vi "Network Streams Chat Window Launcher.vi"() -> ()   [LabVIEW 2020]
uses:
  Chat Window/Chat Window.lvclass
  C:/Program Files (x86)/National Instruments/LabVIEW 2020/vi.lib/ActorFramework/Actor/Actor.lvclass
  Protocols/Network Stream Strategy/Network Stream/Network Stream.lvclass/Network Stream.ctl
  Protocols/Network Stream Strategy/Network Stream Initiator/Network Stream Initiator.lvclass/Network Stream Initiator.ctl
  Chat Window/Chat Window.lvclass/Chat Window.ctl
  Protocols/Network Stream Strategy/Network Stream/Write Buffer Size.vi
  Protocols/Network Stream Strategy/Network Stream/Write Name.vi
  Protocols/Network Stream Strategy/Network Stream Initiator/Network Stream Initiator.lvclass
  C:/justACS/network-endpoints/4.0/Source/Protocols/Network Stream Strategy/Network Stream/Network Stream.lvclass
  C:/justACS/network-endpoints/4.0/Source/Abstract Classes/Message Stream/Message Stream.lvclass
  Protocols/Network Stream Strategy/Netowrk Stream Listener/Network Stream Listener.lvclass
  <vilib>/ActorFramework/Actor/Actor.lvclass
panel:
  in  "Listener Name":string="Bob"
  in  "Address":string="127.0.0.1"
  in  "Initiator Name":string="Fred"
  out "error out":errorcluster
  # "This VI launches two instances of a chat window actor.  The two chat windows launch nested endpoints, which connect via a Network Stream mesage stream.\n\n1.  (Optional)  Specify the IP address for this machine, and the names of the two stream endpoints\n2.  Run this VI.\n3.  Stop the application by closing either chat window.\n\nAF_Debug_Trace is set to TRUE in this project, so you can follow the action with the Desktop Execution Trace Toolkit."
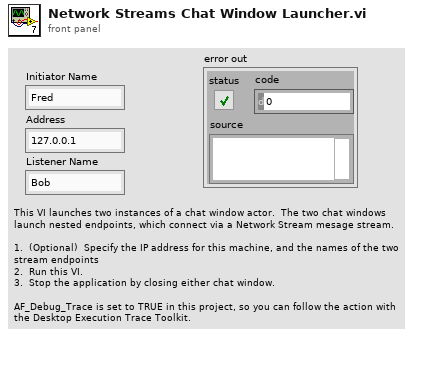
[diagram p1: front panel]
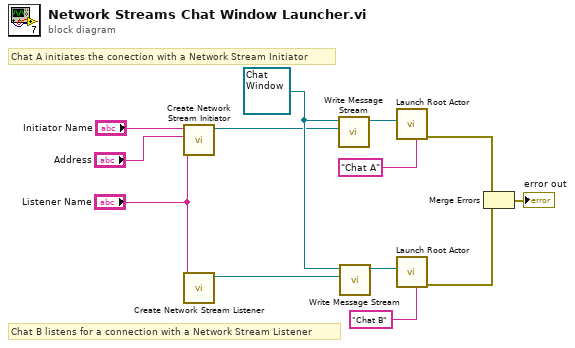
[diagram p0: block diagram]
diagram:
  w13 = refnum<class "Chat Window.lvclass"> refnum ("Chat Window in")
  # "Chat B listens for a connection with a Network Stream Listener"
  # "Chat A initiates the conection with a Network Stream Initiator"
  n1 = call "Create Network Stream Initiator.vi"("Remote Name"="Listener Name", "Remote Address"="Address", "Name"="Initiator Name") -> ("Network Stream Initiator out"=w5:refnum<class "Network Stream Initiator.lvclass">)  [unwired: 8 in]
  n2 = call "Create Network Stream Listener.vi"("Name"="Listener Name") -> ("Network Stream Listener"=w4:refnum<class "Network Stream Listener.lvclass">)  [unwired: 10 in]
  n3 = call "Write Message Stream.vi"("Message Stream"=w5, "Chat Window in"=w13) -> ("Chat Window out"=w12:refnum<class "Chat Window.lvclass">)  [unwired: 9 in]
  n4 = call "Write Message Stream.vi"("Message Stream"=w4, "Chat Window in"=w13) -> ("Chat Window out"=w6:refnum<class "Chat Window.lvclass">)  [unwired: 9 in]
  n5 = call <vilib>:"Launch Root Actor.vi"("Debug Alias"="Chat A", "Actor"=w12) -> ("error out"=w9:errorcluster)  [unwired: 8 in, 1 out]
  n6 = call <vilib>:"Launch Root Actor.vi"("Debug Alias"="Chat B", "Actor"=w6) -> ("error out"=w8:errorcluster)  [unwired: 8 in, 1 out]
  n7 = Merge Errors(w9, w8) -> (→"error out":errorcluster)
